vi "UI elements.vi"() -> ()   [LabVIEW 2025]
uses:
  <vilib>/userDefined/Silver/nirio_resource_slv.ctl
  <vilib>/userDefined/High Color/nirio_resource_hc.ctl
panel:
  in  "NUMERIC 29":dbl
  in  "NUMERIC 28":u64 format="%.0x"
  in  "NUMERIC 27":u16 format="%.0x"
  in  "NUMERIC 26":u8 format="%.0x"
  in  "NUMERIC 25":u16
  in  "NUMERIC 24":u8
  in  "NUMERIC 23":u32 format="%.0x"
  in  "NUMERIC 22":u32
  in  "NUMERIC 21":u64
  out "NUMERIC 20":dbl
  out "NUMERIC 19":u64 format="%.0x"
  out "NUMERIC 18":u16 format="%.0x"
  out "NUMERIC 17":u8 format="%.0x"
  out "NUMERIC 16":u16
  out "NUMERIC 15":u8
  out "NUMERIC 14":u32 format="%.0x"
  out "NUMERIC 13":u32
  out "NUMERIC 12":u64
  out "NUMERIC 11":dbl
  in  "NUMERIC 10":dbl
  out "BOOLEAN 9":bool
  out "BOOLEAN 8":bool
  out "BOOLEAN 7":bool=TRUE
  out "NUMERIC 5":u64 format="%.0x"
  in  "NUMERIC 3":u64 format="%.0x"
  out "NUMERIC":u16 format="%.0x"
  in  "NUMERIC 9":u16 format="%.0x"
  out "NUMERIC":u8 format="%.0x"
  in  "NUMERIC 7":u8 format="%.0x"
  out "NUMERIC":u16
  in  "NUMERIC 8":u16
  out "NUMERIC":u8
  in  "NUMERIC 6":u8
  out "NUMERIC":u32 format="%.0x"
  in  "NUMERIC 4":u32 format="%.0x"
  out "NUMERIC":u32
  in  "NUMERIC 2":u32
  out "BOOLEAN 6":bool
  out "BOOLEAN 5":bool
  out "BOOLEAN 4":bool
  out "BOOLEAN 3":bool
  out "BOOLEAN 2":bool=TRUE
  in  "ENUM 4":enum32{"ITEM0"}(ring)
  in  "RING 4":u32(ring) items=["TERMINATION OFF", "TERMINATION ON"]
  in  "ENUM 3":enum32{"ITEM0"}(ring)
  in  "RING 3":u32(ring) items=["TERMINATION OFF", "TERMINATION ON"]
  in  "ENUM 2":enum32{"ITEM0"}(ring)
  out "PATH TO CONFIG 5":path
  out "PATH TO CONFIG 4":path
  in  "PATH TO CONFIG 3":path
  in  "PATH TO CONFIG 2":path
  in  "XNET DEVICE 2":refnum<k21>
  in  "SWITCH DEVICE 2":refnum<k15>
  in  "RIO DEVICE 2":T1
  in  "STOP 4":bool
  in  "START 2":bool
  in  "STOP 3":bool
  in  "BUTTON 2":bool
  in  "OK":bool
  in  "SETTINGS":enum32{"SETTING1", "SETTING2"}(tab)
  in  "BOOL ARRAY - GREY":bool[][](array[boolean])
  in  "BOOL ARRAY":bool[][](array[boolean])
  in  "SETTINGS":bool
  out "ERROR":bool
  in  "SETTINGS":bool
  in  "INFO":bool
  in  "REMOVE":bool
  in  "MOVE UP":bool
  in  "MOVE DOWN":bool
  in  "ADD":bool
  in  "STOP 2":bool
  out "RESULT":bool
  in  "RESULT":bool
  in  "RING 2":u32(ring) items=["TERMINATION OFF", "TERMINATION ON"]
  in  "STATUS":bool
  in  "COMBO BOX  LONG":string(combo)
  out "ARRAY - STRING":string[](array[string])
  in  "ARRAY - STRING":string[](array[string])
  out "ARRAY - NUMERIC":dbl[](array[numeric])
  in  "ARRAY - NUMERIC":dbl[](array[numeric])
  out "PATH TO CONFIG - SHORT":path
  out "PATH TO CONFIG":path
  in  "PATH TO CONFIG - SHORT":path
  out "STATE MESSAGE 2":string
  in  "STATE MESSAGE":string
  out "LONG STRING":string
  in  "LONG STRING":string
  out "MID STRING":string
  in  "MID STRING":string
  in  "START":bool
  in  "ENUM":enum32{"ITEM0"}(ring)
  in  "RING":u32(ring) items=["ITEM0"]
  out "ERROR":errorcluster
  in  "PATH TO CONFIG":path
  in  "COMBO BOX":string(combo)
  out "SHORT STRING":string
  in  "SHORT STRING":string
  in  "RADIO BUTTON":enum32{"Item 0", "Item 1"}(radio)
  in  "CHECKBOX":bool
  out "BOOLEAN":bool=TRUE
  in  "STOP":bool
  in  "BUTTON":bool
  out "NUMERIC":u64
  in  "NUMERIC":u64
  in  "XNET DEVICE":refnum<k21>
  in  "SWITCH DEVICE":refnum<k15>
  in  "SWITCH DEVICE":refnum<k15>
  in  "SWITCH DEVICE":refnum<k15>
  in  "RIO DEVICE":T1
  in  "RIO DEVICE":T2
  out "DISPLAY":T3(plugin-control)
  # "font 14"
  # "FONT 14"
  # "font 15"
  # "FONT 15"
  # "looks not good but alingned with grid"
  # "control withpout increment"
  # "same visual size as control with increment"
  # "DBL"
  # "HEADLINE1"
  # "U64"
  # "Headline2"
  # "Subtitle"
  # "U64 - hex"
  # "U32"
  # "U32 - hex"
  # "U16"
  # "U16 - hex"
  # "Name \tExample \tValue\nNIBlueBrush \t\t#065FA3\nNIHighlightBrush \t\t#4386B9\nNIBlueMediumAccentBrush \t\t#4386B9\nNIBlueAccentBrush \t\t#82A3D1\nNIHighlightTextBrush \t\t#B3CDE2\nNIHighlightSelectedBrush \t\t#DCE5EC\nNITrueBlackBrush \t\t#000000\nNIBlackBrush \t\t#2B3033\nNIGrayCool36Brush \t\t#4D5359\nNIMediumGrayBrush \t\t#575757\nNIIconGrayBrush \t\t#696E73\nNIGrayBrush \t\t#777B80\nNIDropDownGrayBrush \t\t#82878C\nNIGrayNeutral68Brush \t\t#A9ACAF\nNIBackDropGrayBrush \t\t#B1B4B6\nNIGrayCool81Brush \t\t#C7CCD0\nNIGrayCool88Brush \t\t#D9DEE1\nNIGrayCool90Brush \t\t#DDE2E6\nNIBackgroundBrush \t\t#E0E0E0\nNIWhiteBrush \t\t#EBEBEB\nNIGrayCool92Brush \t\t#E9EBEC\nNIGrayCool94Brush \t\t#EEF0EF\nNIWhiteBlueBrush \t\t#EBF0F5\nNICoolWhiteBrush \t\t#F7F7F7\nNICoolBlue98Brush \t\t#F9FAFC\nNITrueWhiteBrush \t\t#FFFFFF\nNIErrorBrush \t\t#C42126\nNIWarningBrush \t\t#FF8900\nNISuccessBrush \t\t#20B25B\nNIProbeBrush \t\t#006A93\nNIGuidelineBrush \t\t#FC9500\nNIButtonFillBrush \t\t#E9EBEC (Offset: 0%)\n#D9DEE1 (Offset: 40%)"
  # "InstrumentStudio style guide colors\nRED _        NIErrorBrush \t\t#C42126\nORANGE  NIWarningBrush \t\t#FF8900\nGREEN      NISuccessBrush \t\t#20B25B\nBLUE         NIProbeBrush \t\t#006A93\n?                 NIGuidelineBrush \t\t#FC9500\nGrey           NIButtonFillBrush \t\t#E9EBEC (Offset: 0%)\n                                                      #D9DEE1 (Offset: 40%)\n\nrecommended sizes for well alignment\n24\n\n48\n\n72\n\n96\n\n120\n\n144\n\n168\n\n192\n\n216\n\n240"
  # "U8"
  # "U8 - hex"
  # "small button"
  # "large button"
  # "E9EBEC (Offset: 0%)\nD9DEE1"
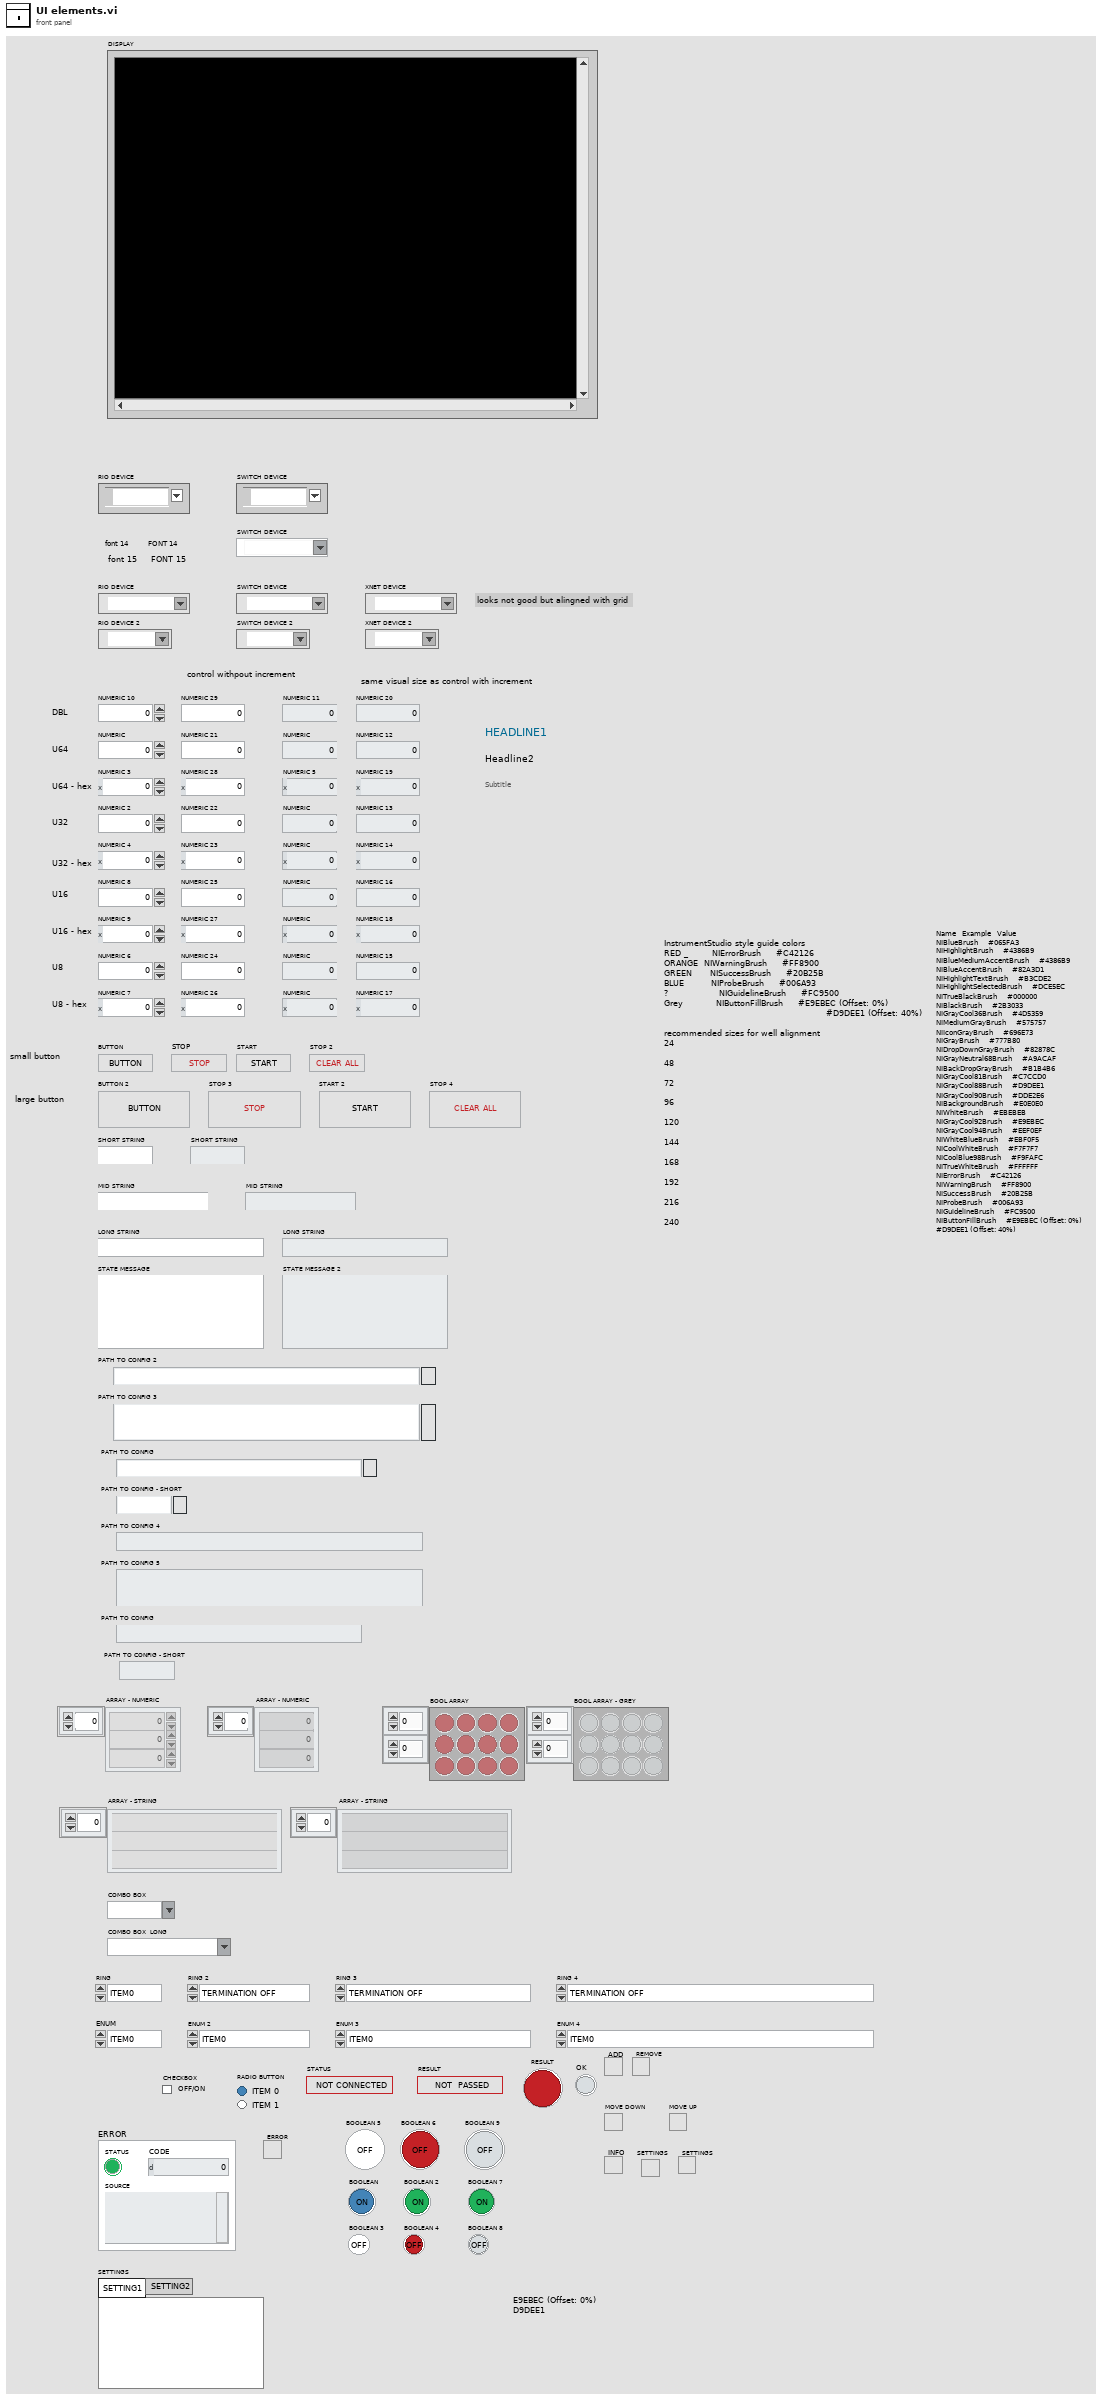
[diagram p1: front panel]
types:
  T1 = typedef "nirio_resource_hc.ctl" = tag
  T2 = typedef "nirio_resource_slv.ctl" = tag
  T3 = typedef "IMAQ Image.ctl" = refnum<image>
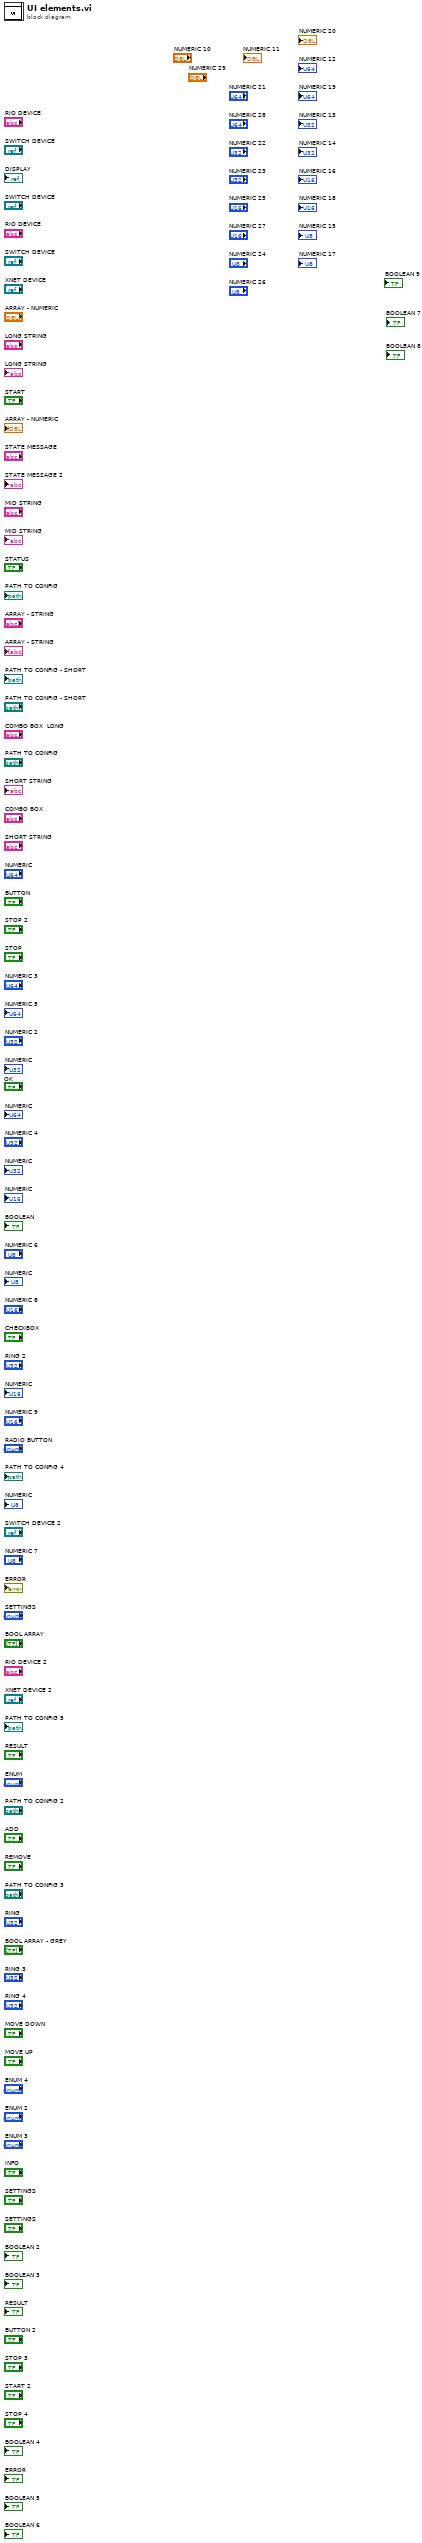
[diagram p0: block diagram]
diagram:
